vi "ValvePos2.vi"(0 "object in":refnum<class "Valve.lvclass">, 5 "error in (no error)":errorcluster) -> (14 "object out":refnum<class "Valve.lvclass">, 19 "error out":errorcluster)   [LabVIEW 2019, in "Valve.lvclass"]
uses:
  Valve.lvclass
  Valve.lvclass/Valve.ctl
panel:
  out "return count":u32
  out "VISA resource name out":refnum<visa-resource-name>
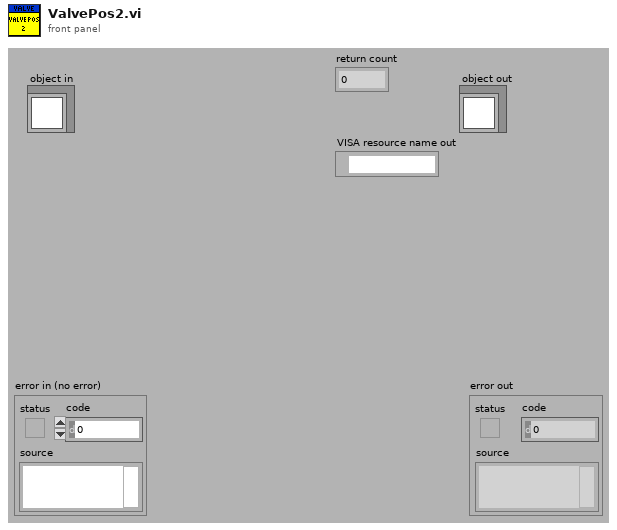
[diagram p1: front panel]
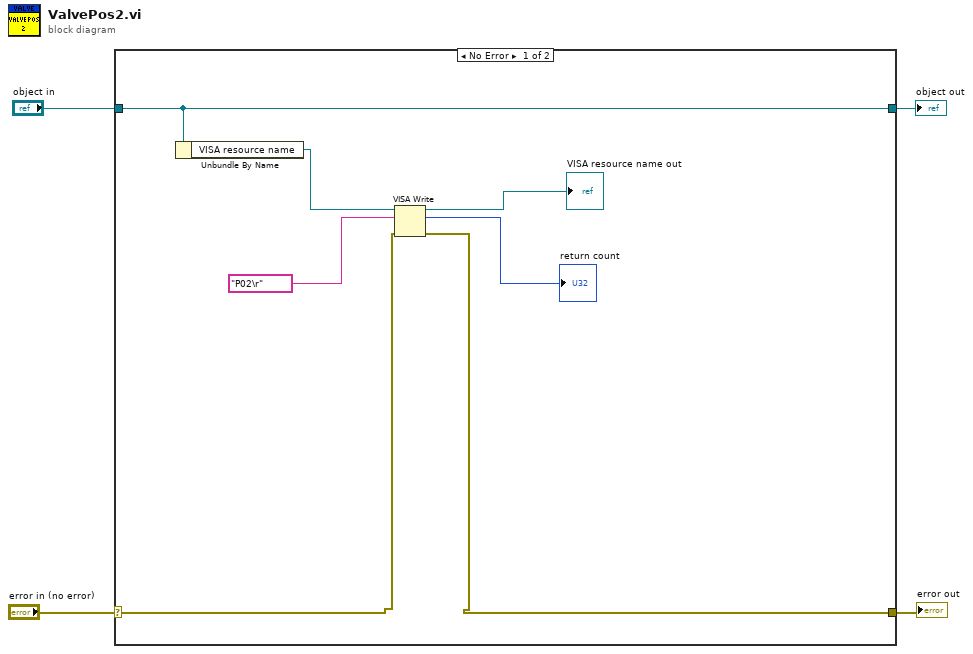
[diagram p0: block diagram]
diagram:
  n1 = case shown="No Error" "error in (no error)" {
    selector: "error in (no error)" -> [w9 w13]
    tunnel: [w8 w13] -> w3
    tunnel: [w11 w12] -> w1
    tunnel: "object in" -> [w11 w12]
    frame No Error {
      n2 = Unbundle By Name(w11) -> ("VISA resource name"=w10:refnum<visa-resource-name>)
      n3 = VISA Write(VISA resource name=w10, write buffer="P02\r", error in (no error)=w9) -> (VISA resource name out=→"VISA resource name out":refnum<visa-resource-name>, return count=→"return count":u32, error out=w8:errorcluster)
    }
    frame Error {
    }
  }
  "error out" <- w3
  "object out" <- w1
